vi "Vms_to_I16Tick.vi"(8 "n":u32=27, 11 "V Velocity [V s-1]":dbl[](array[numeric])=[0.0, 0.0]) -> (0 "V Velocity":i16[](array[numeric]))   [LabVIEW 2023]
uses:
  User_Vi/Settings.vi
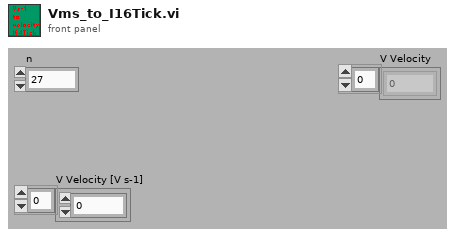
[diagram p1: front panel]
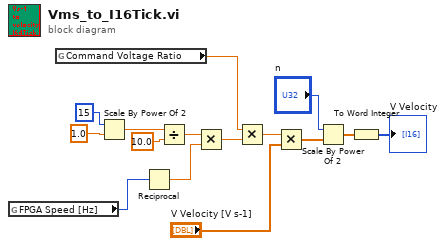
[diagram p0: block diagram]
diagram:
  n1 = global read "Settings.vi" "FPGA Speed [Hz]"() -> (w2:i64)
  n2 = global read "Settings.vi" "Command Voltage Ratio"() -> (w1:dbl)
  n3 = Scale By Power Of 2(n=i16 15, x=1.0) -> (x*2^n=w9:dbl)
  n4 = Reciprocal(x=w2) -> (1/x=w6:dbl)
  n5 = Divide(x=w9, y=10.0 ("Max piezo distance")) -> (x/y=w10:dbl)
  n6 = Multiply(x=w10, y=w6) -> (x*y=w11:dbl)
  n7 = Multiply(x=w1, y=w11) -> (x*y=w3:dbl)
  n8 = Multiply(x=w3, y="V Velocity [V s-1]") -> (x*y=w12:dbl[])
  n9 = Scale By Power Of 2(n="n", x=w12) -> (x*2^n=w5:dbl[])
  n10 = To Word Integer(number=w5) -> (16bit integer=→"V Velocity":i16[])
